vi "Keyboard Navigation.vi"() -> ()   [LabVIEW 2013]
panel:
  in  "Quit":bool
  in  "Save":bool
  in  "Open":bool
  in  "New":bool
  out "Result":string
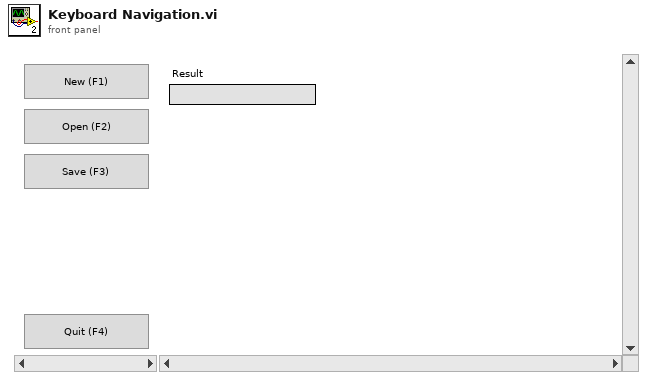
[diagram p1: front panel]
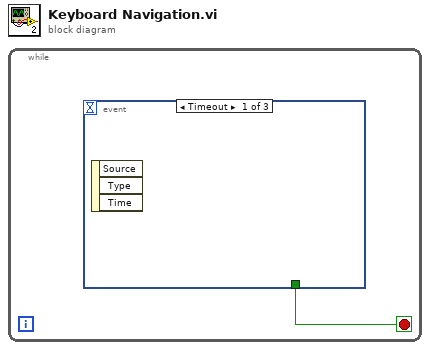
[diagram p0: block diagram]
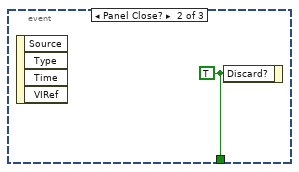
[diagram p2: hidden frame]
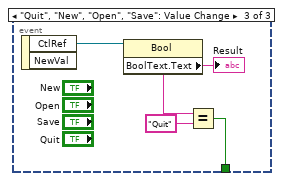
[diagram p3: hidden frame]
diagram:
  n1 = while {
    stop <- w1 stop-if-true
    n2 = event shown="[0] Timeout" {
      selector: _ -> [_ _ _]
      dyn-events: _ -> [_ _ _]
      timeout: _ -> [_ _ _]
      tunnel: [_ w2 w3] -> w1
      event Timeout {
        n3 = event-data() -> ()  [unwired: 1 in, 3 out]
      }
      event Panel Close? {
        w2 = TRUE ("Discard?")
        n4 = event-data() -> ()  [unwired: 1 in, 4 out]
        n5 = event-data("Discard?"=w2) -> ()  [unwired: 1 in, 1 out]
      }
      event "Quit", "New", "Open", "Save": Value Change {
        n6 = event-data() -> ("CtlRef"=w6:refnum<vi>)  [unwired: 1 in, 1 out]
        n7 = property class="Bool"(reference=w6) -> ("BoolText.Text"=w5:string)  [unwired: 1 in, 2 out]
        "Result" <- w5
        n8 = Equal?(x=w5, y="Quit") -> (x = y?=w3:bool)
      }
    }
  }
